vi "Set DHCP Status.vi"(7 "Override?":bool, 8 "Error In":errorcluster, 10 "NIC Mode Override":T1, 11 "NIC Info":T2) -> (0 "Error Out":errorcluster, 3 "NIC Info":T2)   [LabVIEW 2014, in "LMH-LINX.lvlib"]
uses:
  <vilib>/MakerHub/LINX/LMH-LINX.lvlib
  <vilib>/MakerHub/LINX/Private/Utilties/Target Management/NIC Info.ctl
  <vilib>/MakerHub/LINX/Private/Utilties/Target Management/NIC Mode.ctl
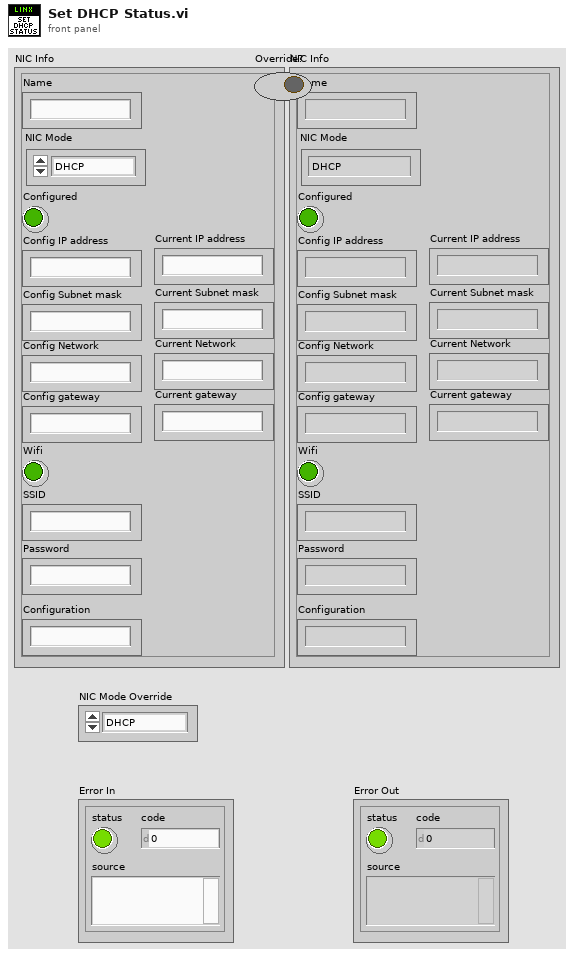
[diagram p1: front panel]
types:
  T1 = typedef "LMH-LINX.lvlib/NIC Mode.ctl" = enum16{"DHCP", "Static", "Loopback"}
  T2 = typedef "LMH-LINX.lvlib/NIC Info.ctl" = cluster{"Name":string, "NIC Mode":T1, "Configured":bool, "Config IP address":string, "Config Subnet mask":string, "Config Network":string, "Config gateway":string, "Wifi":bool, "SSID":string, "Password":string, "Configuration":string, "Current IP address":string, "Current Subnet mask":string, "Current gateway":string, "Current Network":string}
  T3 = enum8{"Enabled", "Disabled", "Disabled and Grayed Out"}
  T4 = typedef "LMH-LINX.lvlib/Network Settings Ctrl Refs.ctl" = cluster{"Hostname":refnum<vi>, "IP address":refnum<vi>, "Subnet mask":refnum<vi>, "Default Gateway":refnum<vi>, "SSID":refnum<vi>, "Password":refnum<vi>, "NIC Status":refnum<vi>, "Network Interface":refnum<vi>, "DCHP":refnum<vi>}
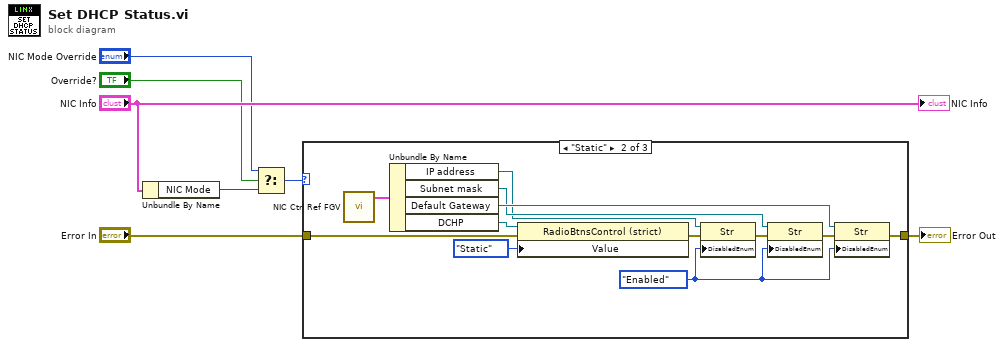
[diagram p0: block diagram]
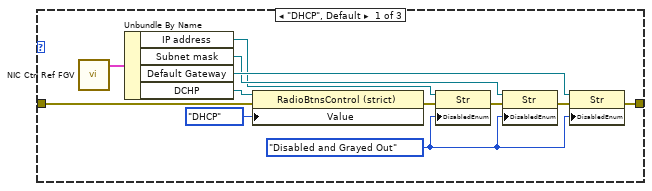
[diagram p2: hidden frame]
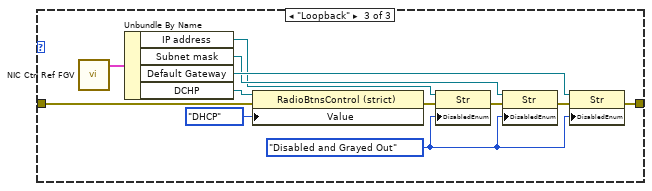
[diagram p3: hidden frame]
diagram:
  n1 = Unbundle By Name("NIC Info") -> ("NIC Mode"=w2:T1)
  n2 = Select(t="NIC Mode Override", s="Override?", f=w2) -> (s? t:f=w1:T1)
  n3 = case shown="\"Static\"" w1 {
    tunnel: "Error In" -> [w14 w26 w38]
    tunnel: [w10 w22 w34] -> w5
    frame "DHCP", Default {
      w19 = T3."Disabled and Grayed Out" ("Disabled")
      n4 = call <vilib>:"NIC Ctrl Ref FGV.vi"() -> ("Network Settings Ctrl Refs"=w15:T4)  [unwired: 4 in]
      n5 = Unbundle By Name(w15) -> ("IP address"=w16:refnum<vi>, "Subnet mask"=w17:refnum<vi>, "Default Gateway"=w18:refnum<vi>, "DCHP"=w9:refnum<vi>)
      n6 = property class="RadioBtnsControl (strict)"(reference=w9, error in=w14, "Value"=enum32{"DHCP", "Static"}."DHCP") -> (error out=w13:errorcluster)  [unwired: 1 out]
      n7 = property class="Str"(reference=w16, error in=w13, "DisabledEnum"=w19) -> (error out=w12:errorcluster)  [unwired: 1 out]
      n8 = property class="Str"(reference=w17, error in=w12, "DisabledEnum"=w19) -> (error out=w11:errorcluster)  [unwired: 1 out]
      n9 = property class="Str"(reference=w18, error in=w11, "DisabledEnum"=w19) -> (error out=w10:errorcluster)  [unwired: 1 out]
    }
    frame "Static" {
      w31 = T3."Enabled" ("Disabled")
      n10 = call <vilib>:"NIC Ctrl Ref FGV.vi"() -> ("Network Settings Ctrl Refs"=w27:T4)  [unwired: 4 in]
      n11 = Unbundle By Name(w27) -> ("IP address"=w28:refnum<vi>, "Subnet mask"=w29:refnum<vi>, "Default Gateway"=w30:refnum<vi>, "DCHP"=w21:refnum<vi>)
      n12 = property class="RadioBtnsControl (strict)"(reference=w21, error in=w26, "Value"=enum32{"DHCP", "Static"}."Static") -> (error out=w25:errorcluster)  [unwired: 1 out]
      n13 = property class="Str"(reference=w28, error in=w25, "DisabledEnum"=w31) -> (error out=w24:errorcluster)  [unwired: 1 out]
      n14 = property class="Str"(reference=w29, error in=w24, "DisabledEnum"=w31) -> (error out=w23:errorcluster)  [unwired: 1 out]
      n15 = property class="Str"(reference=w30, error in=w23, "DisabledEnum"=w31) -> (error out=w22:errorcluster)  [unwired: 1 out]
    }
    frame "Loopback" {
      w43 = T3."Disabled and Grayed Out" ("Disabled")
      n16 = call <vilib>:"NIC Ctrl Ref FGV.vi"() -> ("Network Settings Ctrl Refs"=w39:T4)  [unwired: 4 in]
      n17 = Unbundle By Name(w39) -> ("IP address"=w40:refnum<vi>, "Subnet mask"=w41:refnum<vi>, "Default Gateway"=w42:refnum<vi>, "DCHP"=w33:refnum<vi>)
      n18 = property class="RadioBtnsControl (strict)"(reference=w33, error in=w38, "Value"=enum32{"DHCP", "Static"}."DHCP") -> (error out=w37:errorcluster)  [unwired: 1 out]
      n19 = property class="Str"(reference=w40, error in=w37, "DisabledEnum"=w43) -> (error out=w36:errorcluster)  [unwired: 1 out]
      n20 = property class="Str"(reference=w41, error in=w36, "DisabledEnum"=w43) -> (error out=w35:errorcluster)  [unwired: 1 out]
      n21 = property class="Str"(reference=w42, error in=w35, "DisabledEnum"=w43) -> (error out=w34:errorcluster)  [unwired: 1 out]
    }
  }
  "Error Out" <- w5
  "NIC Info" <- "NIC Info"
